vi "读测量文件.vi"() -> ()   [LabVIEW 2010]
uses:
  Instance           1 18Saved   读测量文件 .vi
panel:
  out "波形图":dynamicdata(graph)
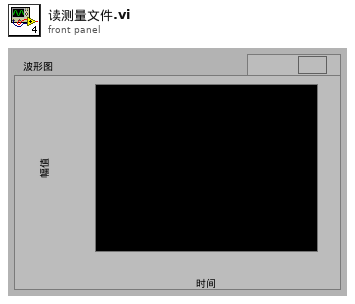
[diagram p1: front panel]
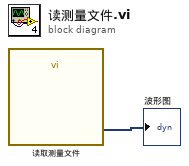
[diagram p0: block diagram]
diagram:
  n1 = call "读取测量文件"() -> ("Signals"=→"波形图":dynamicdata)  [unwired: 6 in, 5 out]
